vi "Configure Wide Limit Test.vi"(0 "VISA resource name":refnum<visa-resource-name>, 1 "Enable Wide Limit Test (F: Disable)":bool, 5 "Configure Wide Upper Limit (1)":dbl=1.0, 7 "Configure Wide Lower Limit (-1)":dbl=-1.0, 11 "error in (no error)":errorcluster, 12 "Wide Upper Limit Fail Bit Pattern (15)":u16=15, 13 "Wide Lower Limit Fail Bit Pattern (15)":u16=15) -> (4 "VISA resource name out":refnum<visa-resource-name>, 15 "error out":errorcluster)   [LabVIEW 2021, in "Keithley 648X Series.lvlib"]
doc: "Configures the wide limit of the limit test. The instrument assumes the wide limit wholly contains the narrow limit.\n\n<b>Note:</b>\nThis VI is part of the component handler interfacing VIs."
uses:
  <instrlib>/Keithley 648X Series/Keithley 648X Series.lvlib
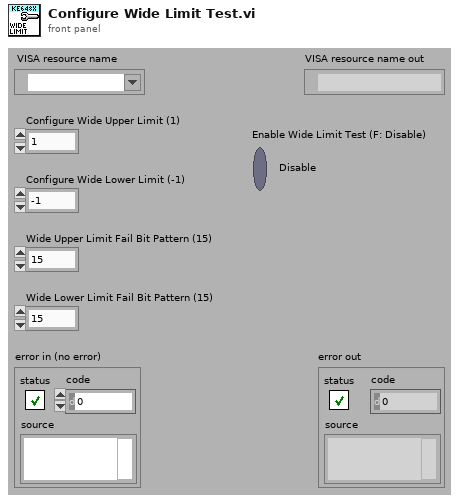
[diagram p1: front panel]
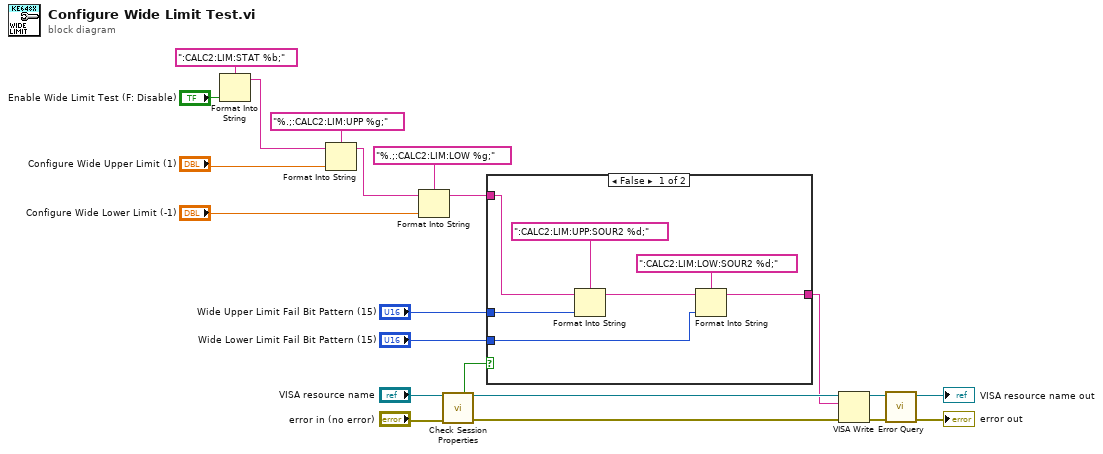
[diagram p0: block diagram]
diagram:
  n1 = Format Into String(format string=":CALC2:LIM:STAT %b;", "Enable Wide Limit Test (F: Disable)") -> (resulting string=w13:string)  [unwired: 2 in, 1 out]
  n2 = Format Into String(format string="%.;:CALC2:LIM:UPP %g;", initial string=w13, "Configure Wide Upper Limit (1)") -> (resulting string=w12:string)  [unwired: 1 in, 1 out]
  n3 = Format Into String(format string="%.;:CALC2:LIM:LOW %g;", initial string=w12, "Configure Wide Lower Limit (-1)") -> (resulting string=w2:string)  [unwired: 1 in, 1 out]
  n4 = call <instrlib>:"Check Session Properties.vi"("VISA resource name"="VISA resource name", "error in (no error)"="error in (no error)") -> ("Model 6485"=w5:bool, "VISA resource name out"=w9:refnum<visa-resource-name>, "error out"=w8:errorcluster)  [unwired: 10 in, 1 out]
  n5 = case shown="False" w5 {
    tunnel: "Wide Upper Limit Fail Bit Pattern (15)" -> [w26 _]
    tunnel: "Wide Lower Limit Fail Bit Pattern (15)" -> [w24 _]
    tunnel: w2 -> [w27 w29]
    tunnel: [w22 w29] -> w1
    frame False {
      n6 = Format Into String(format string=":CALC2:LIM:UPP:SOUR2 %d;", initial string=w27, w26) -> (resulting string=w23:string)  [unwired: 1 in, 1 out]
      n7 = Format Into String(format string=":CALC2:LIM:LOW:SOUR2 %d;", initial string=w23, w24) -> (resulting string=w22:string)  [unwired: 1 in, 1 out]
    }
    frame True {
      # "Model 6485 doesn't output fail bit patterns"
    }
  }
  n8 = VISA Write(VISA resource name=w9, write buffer=w1, error in (no error)=w8) -> (VISA resource name out=w19:refnum<visa-resource-name>, error out=w18:errorcluster)  [unwired: 1 out]
  n9 = call <instrlib>:"Error Query.vi"("error in (no error)"=w18, "VISA resource name"=w19) -> ("error out"=→"error out":errorcluster, "VISA resource name out"=→"VISA resource name out":refnum<visa-resource-name>)  [unwired: 6 in, 2 out]
